vi "Send Redraw Configuration.vi"(8 "error in (no error)":errorcluster, 11 "AssertEngine in":refnum<class "AssertEngine.lvclass">) -> (0 "error out":errorcluster)   [LabVIEW 2016, in "AssertEngine.lvlib" / "AssertEngine.lvclass"]
uses:
  AssertEngine.lvclass
  UserInterface/UserInterface/Sort Configuration.ctl
  AssertEngine.lvclass/AssertEngine.ctl
  UserInterface/UserInterface Messages/Draw Assert Data Msg/Draw Assert Data Msg.lvclass/Draw Assert Data Msg.ctl
  <vilib>/ActorFramework/Message Enqueuer/Message Enqueuer.lvclass/Message Enqueuer.ctl
  <vilib>/ActorFramework/Message Enqueuer/Enqueue.vi
  UserInterface/UserInterface Messages/Draw Assert Data Msg/Draw Assert Data Msg.lvclass
  C:/Program Files/National Instruments/LabVIEW 2016/vi.lib/ActorFramework/Message/Message.lvclass
  <vilib>/ActorFramework/Message Priority Queue/Priority Enqueue.vi
  UserInterface/UserInterface/UserInterface.lvclass
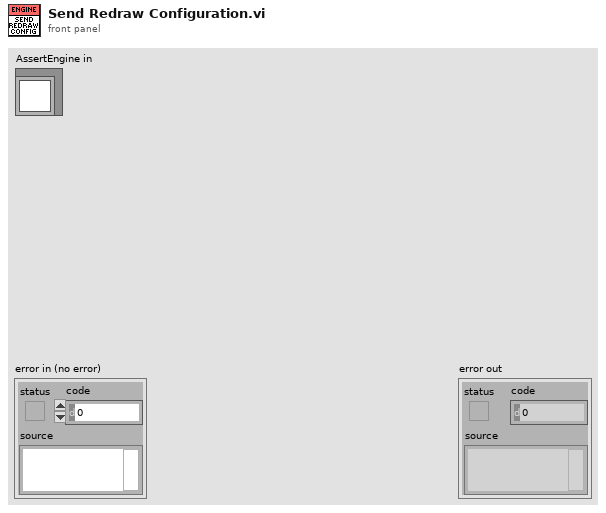
[diagram p1: front panel]
types:
  T1 = typedef "UserInterface.lvlib/UserInterface.lvclass/Sort Configuration.ctl" = cluster{"Column to Sort By":u32, "Order":enum16{"ascending", "descending"}}
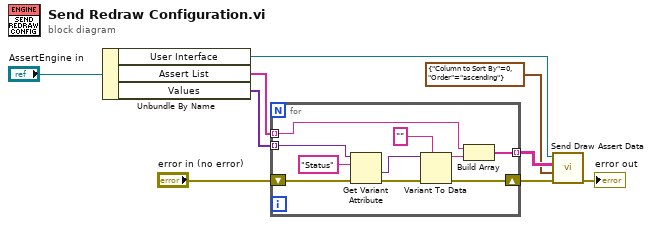
[diagram p0: block diagram]
diagram:
  n1 = Unbundle By Name("AssertEngine in") -> ("User Interface"=w7:refnum<class "Message Enqueuer.lvclass">, "Assert List"=w4:string[], "Values"=w6:variant[])
  n2 = for {
    tunnel: w6 -> [w19] mode=indexing
    shift-right: [w10] -> w2
    shift-left: "error in (no error)" -> [w17]
    tunnel: w4 -> [w13] mode=indexing
    tunnel: [w11] -> w3 mode=indexing
    n3 = Get Variant Attribute(Variant=w19, name="Status", error in=w17) -> (value=w15:variant, error out=w16:errorcluster)  [unwired: 1 in, 2 out]
    n4 = Variant To Data(error in=w16, type="" ("name"), Variant=w15) -> (data=w12:string, error out=w10:errorcluster)
    n5 = Build Array(w13, w12) -> (w11:string[])
  }
  n6 = call "Send Draw Assert Data.vi"("error in (no error)"=w2, "Sort Configuration"=T1 {"Column to Sort By"=0, "Order"=enum."ascending"}, "Assert Data"=w3, "Message Enqueuer"=w7) -> ("error out"=→"error out":errorcluster)  [unwired: 6 in, 1 out]
